vi "item amount.vi"() -> ()   [LabVIEW 2025]
panel:
  out "Item amount":u32
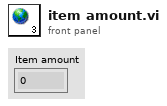
[diagram p1: front panel]
diagram:
